vi "Global variable.vi"   [LabVIEW 2024]
uses:
  Global 4.vi
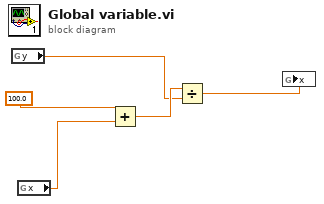
[diagram p0: block diagram]
diagram:
  n1 = global read "Global 4.vi" "y"() -> (w1:dbl)
  n2 = global read "Global 4.vi" "x"() -> (w3:dbl)
  n3 = Add(x=100.0, y=w3) -> (x+y=w2:dbl)
  n4 = Divide(x=w2, y=w1) -> (x/y=w4:dbl)
  n5 = global write "Global 4.vi" "x"(w4) -> ()
